vi "CloseLeonardoAsJoystick.vi"(8 "error in (no error)":errorcluster, 11 "Refnum in":refnum<k1>) -> ()   [LabVIEW 2014]
doc: "Close reference to Leonardo joystick"
uses:
  <vilib>/Utility/inputDevices.llb/closeJoystick.vi
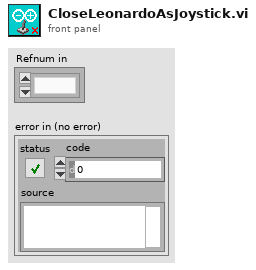
[diagram p1: front panel]
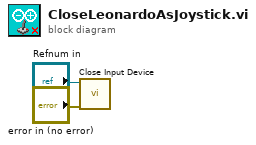
[diagram p0: block diagram]
diagram:
  n1 = call-poly <vilib>:"Close Input Device.vi"("error in (no error)"="error in (no error)", "device ID"="Refnum in") -> ()  [unwired: 8 in, 1 out]
